vi "display waveforms.vi"() -> ()   [LabVIEW 2013]
uses:
  Controls/waveform display.ctl
panel:
  in  "Array 2":T1[][](array[typedef])
  in  "Array":waveform(dbl)[](array[waveform])
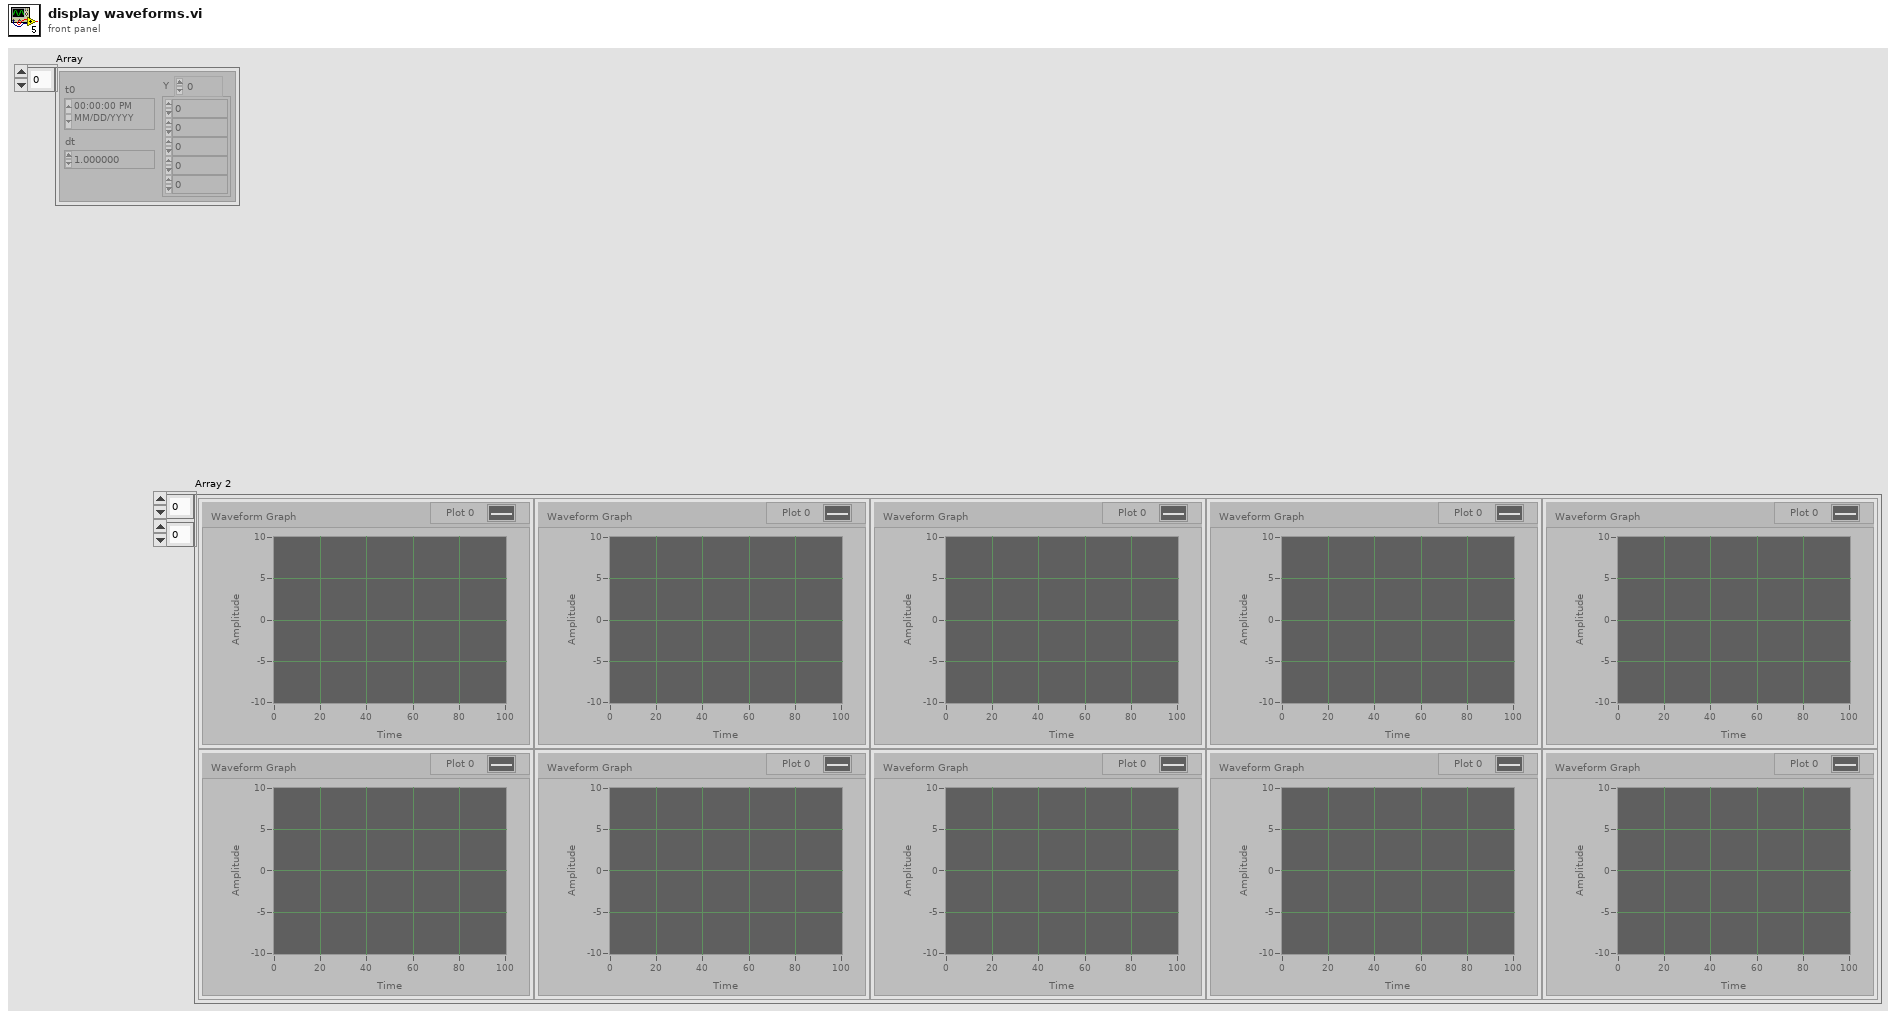
[diagram p1: front panel]
types:
  T1 = typedef "waveform display.ctl" = cluster{"Waveform Graph":dbl[]}
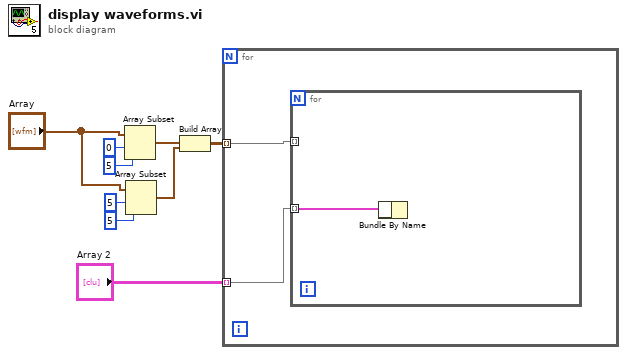
[diagram p0: block diagram]
diagram:
  n1 = Array Subset(array="Array", index=0, length=5) -> (w4:waveform(dbl)[])
  n2 = Array Subset(array="Array", index=5, length=5) -> (w3:waveform(dbl)[])
  n3 = Build Array(w4, w3) -> (w2:waveform(dbl)[][])
  n4 = for {
    tunnel: w2 -> [w11] mode=indexing
    tunnel: "Array 2" -> [w10] mode=indexing
    n5 = for {
      tunnel: w11 -> [_] mode=indexing
      tunnel: w10 -> [w12] mode=indexing
      n6 = Bundle By Name(w12) -> ()  [unwired: 1 in, 1 out]
    }
  }
